vi "P10.vi"() -> ()   [LabVIEW 2018]
uses:
  <vilib>/userdefined/High Color/IMAQdx.ctl
  <vilib>/vision/driver/IMAQdx.llb/IMAQdx Acquisition Mode.ctl
  <vilib>/vision/driver/NI_Vision_Acquisition_Software.lvlib
panel:
  out "error out":errorcluster
  out "Image":T1(plugin-control)
  in  "stop":bool
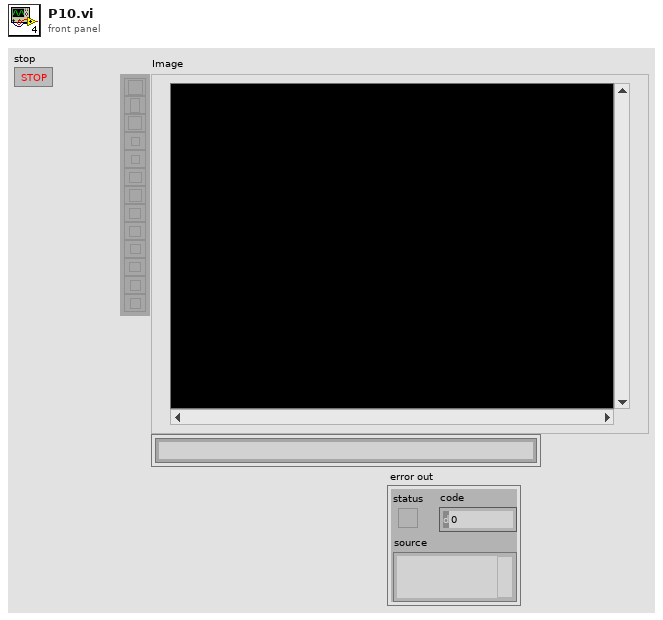
[diagram p1: front panel]
types:
  T1 = typedef "IMAQ Image.ctl" = refnum<image>
  T2 = typedef "Image Type" = u32
  T3 = typedef "NI_Vision_Acquisition_Software.lvlib/IMAQdx Acquisition Mode.ctl" = enum32{"One Shot", "Continuous"}
  T4 = typedef "IMAQdx.ctl" = refnum<k21>
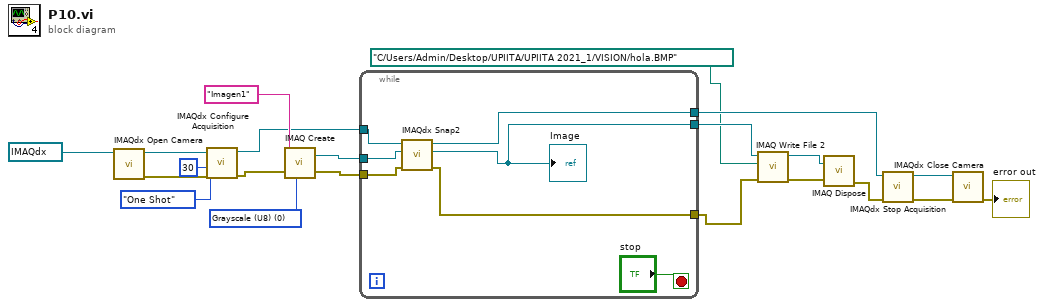
[diagram p0: block diagram]
diagram:
  w15 = T2 0 items=["Grayscale (U8)", "Grayscale (I16)", "Grayscale (SGL)", "Complex (CSG)", "RGB (U32)", "HSL (U32)", "RGB (U64)", "Grayscale (U16)"] ("Image Type")
  n1 = call <vilib>:"IMAQdx Open Camera.vi"("Session In"=T4 "cam0") -> ("error out"=w19:errorcluster, "Session Out"=w20:T4)  [unwired: 9 in]
  n2 = call <vilib>:"IMAQdx Configure Acquisition.vi"("error in"=w19, "Number of Buffers"=u32 30, "Continuous?"=IMAQdx_Acquisition_Mode."One Shot", "Session In"=w20) -> ("error out"=w14:errorcluster, "Session Out"=w13:T4)  [unwired: 6 in]
  n3 = call "IMAQ Create"("Image Name"="Imagen1", "Image Type"=w15, "error in (no error)"=w14) -> ("New Image"=w11:T1, "error out"=w12:errorcluster)  [unwired: 2 in]
  n4 = while {
    tunnel: w13 -> [w25]
    tunnel: w12 -> [w26]
    tunnel: w11 -> [w27]
    tunnel: [w24] -> w7
    tunnel: [w23] -> w3
    tunnel: [w22] -> w2
    stop <- "stop" stop-if-true
    n5 = call <vilib>:"IMAQdx Snap2.vi"("error in"=w26, "Image In"=w27, "Session In"=w25) -> ("error out"=w22:errorcluster, "Image Out"=w23:T1, "Session Out"=w24:T4)  [unwired: 6 in]
    "Image" <- w23
  }
  n6 = call-poly "IMAQ Write File 2"("error in (no error)"=w2, "File Path"=path "C:/Users/Admin/Desktop/UPIITA/UPIITA 2021_1/VISION/hola.BMP", "Image"=w3) -> ("error out"=w4:errorcluster, "Image Out (duplicate)"=w5:T1)  [unwired: 7 in]
  n7 = call "IMAQ Dispose"("Image"=w5, "error in (no error)"=w4) -> ("error out"=w10:errorcluster)  [unwired: 4 in]
  n8 = call <vilib>:"IMAQdx Stop Acquisition.vi"("error in"=w10, "Session In"=w7) -> ("error out"=w9:errorcluster, "Session Out"=w6:T4)  [unwired: 8 in]
  n9 = call <vilib>:"IMAQdx Close Camera.vi"("error in"=w9, "Session In"=w6) -> ("error out"=→"error out":errorcluster)  [unwired: 9 in]
